vi "end_of_cell.vi"(1 "buffer in":string) -> (0 "Boolean":bool)   [LabVIEW 2016]
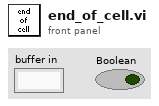
[diagram p1: front panel]
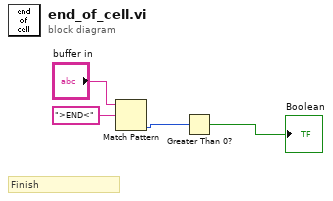
[diagram p0: block diagram]
diagram:
  # "Finish"
  n1 = Match Pattern(string="buffer in", regular expression=">END<") -> (offset past match=w2:i32)  [unwired: 1 in, 3 out]
  n2 = Greater Than 0?(x=w2) -> (x > 0?=→"Boolean":bool)
